vi "Write Analog Input Waveform Data Msg.vi"(8 "error in (no error)":errorcluster, 10 "DAQmx Actor Interface.lvlib:Analog Input Waveform Data Msg.lvclass":refnum<class "Analog Input Waveform Data Msg.lvclass">, 11 "Analog Reader in":refnum<class "Analog Reader.lvclass">) -> (0 "error out":errorcluster, 3 "Analog Reader out":refnum<class "Analog Reader.lvclass">)   [LabVIEW 2024]
uses:
  Analog Reader.lvclass
  DAQmx Actor Interface/Analog Input Waveform Data Messages/Analog Input Waveform Data Msg/Analog Input Waveform Data Msg.lvclass
  Analog Reader.lvclass/Analog Reader.ctl
  C:/Users/uspoaotto/OneDrive - Oregon Tool/Desktop/working copies/DAQmxActor/src/DAQmx Actor/DAQmx Actor/DAQmx Actor.lvclass
  C:/Program Files (x86)/National Instruments/LabVIEW 2024/vi.lib/ActorFramework/Actor/Actor.lvclass
  C:/Users/uspoaotto/OneDrive - Oregon Tool/Desktop/working copies/DAQmxActor/src/DAQmx Actor/Analog Reader/Analog Reader.lvclass
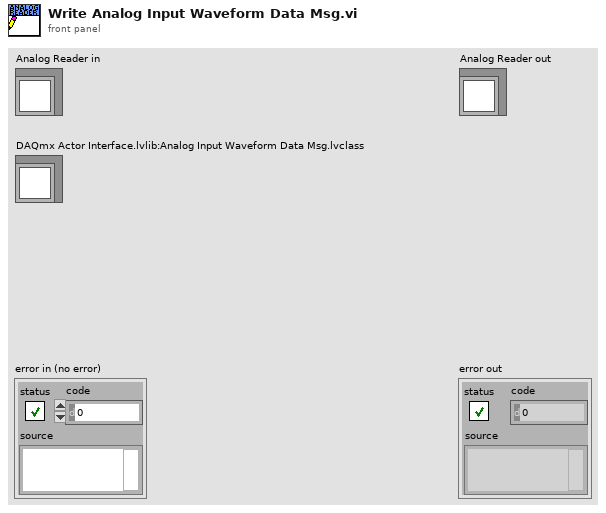
[diagram p1: front panel]
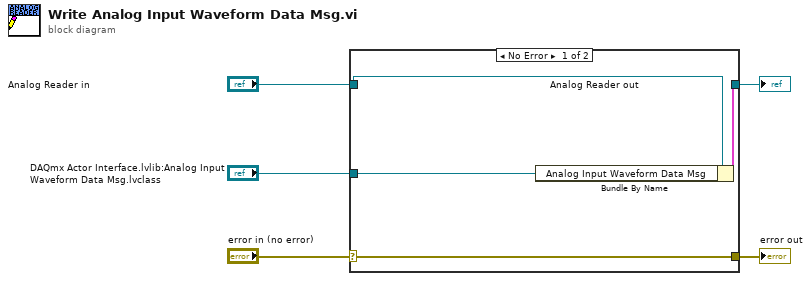
[diagram p0: block diagram]
diagram:
  n1 = case shown="No Error" "error in (no error)" {
    selector: "error in (no error)" -> [w9 w10]
    tunnel: [w9 w10] -> w4
    tunnel: [w7 w11] -> w2
    tunnel: "Analog Reader in" -> [w8 w11]
    tunnel: "DAQmx Actor Interface.lvlib:Analog Input Waveform Data Msg.lvclass" -> [w6 _]
    frame No Error {
      n2 = Bundle By Name(cluster=w8, "Analog Input Waveform Data Msg"=w6) -> (w7:cluster{})
    }
    frame Error {
    }
  }
  "error out" <- w4
  "Analog Reader out" <- w2
